vi "Big_LED_control.vi"() -> ()   [LabVIEW 2018]
uses:
  AT lib/AmateurStepperMotor.dll
  <instrlib>/niDMM/nidmm.llb/niDMM Function.ctl
  <instrlib>/niDMM/nidmm.llb/niDMM Resolution in Digits.ctl
  <instrlib>/niDCPower/nidcpower.llb/niDCPower Measurement Type.ctl
  <vilib>/Instr/_visa.llb/VISA Configure Serial Port (Instr).vi
  <instrlib>/niDMM/nidmm.llb/niDMM Configure Measurement Digits.vi
panel:
  out "IsOpen":bool
  out "Enum":enum16{"Exit", "4", "Промер", "2", "1"}(ring)
  in  "Tab Control":T1(tab)=enum."Сила света"
  in  "POWER":bool
  in  "Стоп":bool=TRUE
  in  "Resource Name":refnum<k15>="PXI1Slot2" caption="Источник питания"
  in  "Амперметр":refnum<k15>="PXI1Slot4" caption="NI DMM 1"
  in  "V_MB, V":dbl=5.0 caption="voltage level" format="%_6p"
  in  "curlim_V_MB, A":dbl=0.3 caption="current limit" format="%_6p"
  in  "curlim_V_RESERVE, A":dbl=0.1 caption="current limit" min=0.01 format="%_6p"
  out "currentmes_V_MB, A":dbl=-0.001986406197333734 caption="measurement" format="%_6g"
  out "currentmes_V_RESERVE, A":dbl=4.286668577189643e-07 caption="measurement" format="%_6g"
  in  "V_RESERVE, V":dbl caption="voltage level" format="%_6p"
  out "chart_2":dbl(graph)=4.286668577189643e-07
  out "chart_0":dbl(graph)=-0.001986406197333734 caption="Waveform Chart 5"
  in  "curlim_V_LED, A":dbl=0.01 caption="current limit" min=0.01 format="%_6p"
  in  "V_LED, V":dbl=2.000000000000001 caption="voltage level" format="%_6p"
  out "chart_1":dbl(graph)=9.464711192498274e-07 caption="Waveform Chart 5"
  out "currentmes_V_LED, A":dbl=9.464711192498274e-07 caption="measurement" format="%_6g"
  in  "NI DMM 1 Current Range 3":string(combo)="1" caption="Range"
  in  "NI DMM 1 units 3":string(combo)="1000" caption="Units"
  out "Current Char":dbl(graph)=0.008323229849338531
  out "Current":dbl=0.008323229849338531 format="%_6g"
  in  "Arduino":refnum<visa-resource-name>="COM14"
  in  "Сегменты":bool[](array[boolean])=[FALSE, FALSE, FALSE, FALSE, FALSE, FALSE, FALSE, FALSE, FALSE, FALSE, FALSE, FALSE, FALSE, FALSE, FALSE, FALSE, FALSE, FALSE]
  in  "Вольтметр":refnum<k15>="PXI1Slot5" caption="NI DMM 1"
  in  "NI DMM 1 Voltage Range 4":string(combo)="-1" caption="Range"
  out "Voltage Char":dbl(graph)=nan
  in  "NI DMM 1 units 4":string(combo)="1" caption="Units"
  out "Voltage":dbl=nan format="%_6g"
  out "Тип индикатора":string="Anode"
  in  "set pos":bool
  in  "new pos":dbl
  in  "Промер":bool caption="Промер сегмента"
  in  "Ophir 1 Info":u16(ring)=1 caption="Info" items=["Device : JUNO; s/n:903793", "Head : PD300R-3W   ; s/n:779628"]
  out "Ophir 1 Initialization":bool=TRUE caption="Initialization"
  out "Position":dbl
  out "Готово":bool
  in  "Стоп GoTo":bool
  in  "Погнали!":bool
  in  "Speed":dbl=1000.0
  in  "StepDivisor":i32(ring)=8 items=["D1"=1, "D2"=2, "D4"=4, "D8"=8, "D16"=16, "D32"=32]
  in  "StepMultiplicationFactor":dbl=1.0
  in  "Ophir 1 Wait":u32=100 caption="Wait"
  in  "Ophir 1 Clear":bool caption="Clear"
  out "Ophir 1 MAX":dbl=0.060000000000000005 caption="MAX" format="%#_5g"
  out "Ophir 1 Optical Power":dbl=0.060000000000000005 caption="Power" format="%#_4g"
  out "Ophir 1 Over Range":bool caption="Over Range"
  in  "Ophir 1 units":string(combo)="1000" caption="Units"
  in  "HoldOn":bool
  in  "AccelerationTime, s":dbl
  in  "DecelerationTime, s":dbl
  out "Ophir 1 Char":dbl(graph)=0.060000000000000005
  in  "Go To":dbl
  in  "wave_lenght":string="600"
  in  "Port Name":string="COM1"
  in  "measure path":path=path "D:/NI LabVIEW/MultiOpto/MultiOpto_1.2/Logs/SEL"
  in  "Сегмент":string="-" caption="Введи сегмент"
  in  "Температура":string="-" caption="Введи температуру"
  out "Образец №":string="0"
  in  "milliseconds to wait":u32=1000
  out "Разряд":dbl
  out "+/-":bool
  out "Power off":bool=TRUE
  in  "Ophir 1 error in (no error)":errorcluster caption="error in (no error)"
  out "Ophir 1 error out":errorcluster caption="error out"
  in  "Ophir 1 Select Communication Protocol":u16(ring) caption="Select Communication Protocol" items=["USB", "RS232", "GPIB"]
  in  "Ophir 1 Port Number (default 2)":i16=1 caption="Port Number (default 2)" min=0 max=20
  in  "Ophir 1 GPIB Address (10)":string="10" caption="GPIB Address (10)"
  out "Ophir 1 Real Optical Power":dbl=6e-05 format="%.6e"
  in  "Ophir 1 Baud Rate (3:9600)":i16(ring)=3 caption="Baud Rate (3:9600)" items=["300", "1200", "4800", "9600", "19200", "38400"]
  out "Ophir 1 dup Visa Session":refnum<visa-resource-name>="USB0::0x0BD3::0x0777::NI-VISA-40004::RAW" caption="dup Visa Session"
  in  "Ophir 1 usb channel":i16 caption="usb channel"
  in  "Command":string="Anode"
  in  "Записать":bool
  out "measure output file refnum":refnum<file>
  out "Device Response":string="*\n"
  out "Voltage, V":dbl=nan caption="Measurement" format="%.5f"
  out "Current, A":dbl=8.323229849338531e-06 caption="Measurement" format="%.5f"
  # "V_MB 5 В\nогрничение 300 м\n\nV_LED 2,1 В\nограничение 200 м"
  # "единицы мА\nrange 1 А"
  # "единицы В\nrange AUTO"
  # "24.063\n\n     I          U\n20 мА  1.3 В\n20 мА  1.4 В\n 7 мА   1.15 В"
  # "24.064\n\n     I          U\n10 мА  2 В\n10 мА  2.15 В\n 7 мА   1.9 В"
  # "Р1:  +25°C\nР2:  - 60°C\nР3:  +85°C"
  # "j"
  # "c"
  # "d"
  # "e"
  # "g"
  # "h"
  # "a"
  # "b"
  # "f"
  # "k"
  # "L"
  # "m"
  # "n"
  # "p"
  # "dp"
  # "all"
  # "необходимо выдерживать 1 с между нажатиями кнопок"
  # "Шаговик"
  # "Офир"
  # "это значение абсолютное"
  # "0. ввести номер образца\n1. включить нужный сегмент\n2. ввести его в поле справа\n3. вести температуру в поле слева\n4. нажать кнопку \"промер сегмента\""
  # "Введи ->"
  # "\"опрашивать кнопки не чаще, чем раз в секунду. сейчас кликать можно чаще, они загорятся, но ничего не произойдет\""
  # "Офир"
  # "автоматизировать подбор напряжения по известному максимальному напряжению и току. ОС по току сегмента"
  # "регклировка суммарного тока через индикатор"
  # "регулировать ток в зависимости от температуры.\nс ростом температуры растет ток.\nпид-регулятор??"
  # "1. каждый сегмент включаем по отдельности, резистором постраиваем ток до 10 мА\n2. напряжение V_LED при этом не меняется\n3. в такоом положении промеряем сегменты по отдельности\n4. для промера всего индикатора сразу подстраиваем напряжение при неизменном положении резисторов\n5. ток всех индикаторов = ток одного сегмента (10 мА) * число сегментов (15)\n6. добиваемся этого увеличением V_LED"
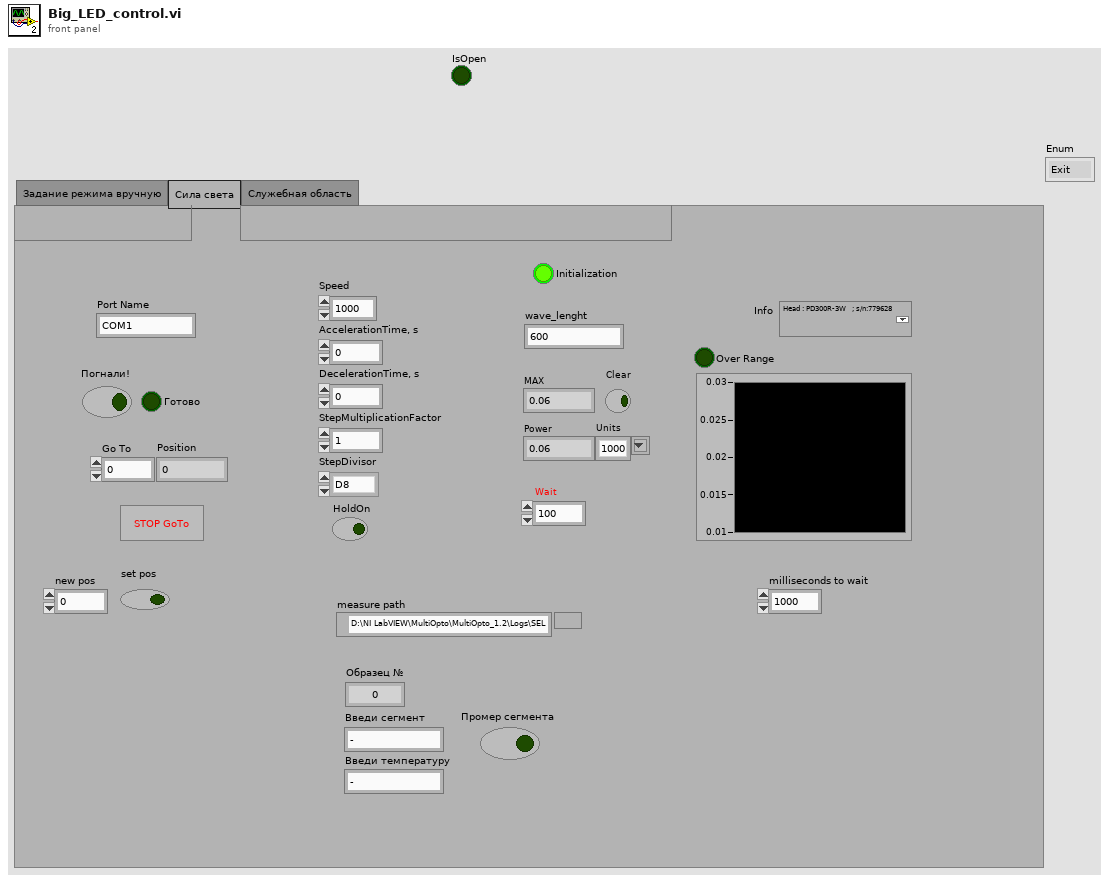
[diagram p1: front panel]
types:
  T1 = enum32{"Задание режима вручную", "Сила света", "Служебная область"}
  T2 = enum16{"open", "replace", "create", "open or create", "replace or create", "replace or create with confirmation"}
  T3 = typedef "niDCPower Measurement Type.ctl" = i32
  T4 = typedef "niDMM Function.ctl" = enum16{"DC Volts", "AC Volts", "DC Current", "AC Current", "2-wire Resistance", "4-wire Resistance", "Diode", "Frequency", "Period", "AC Volts DC Coupled", "Capacitance", "Inductance", "Temperature"}
  T5 = typedef "niDMM Resolution in Digits.ctl" = dbl
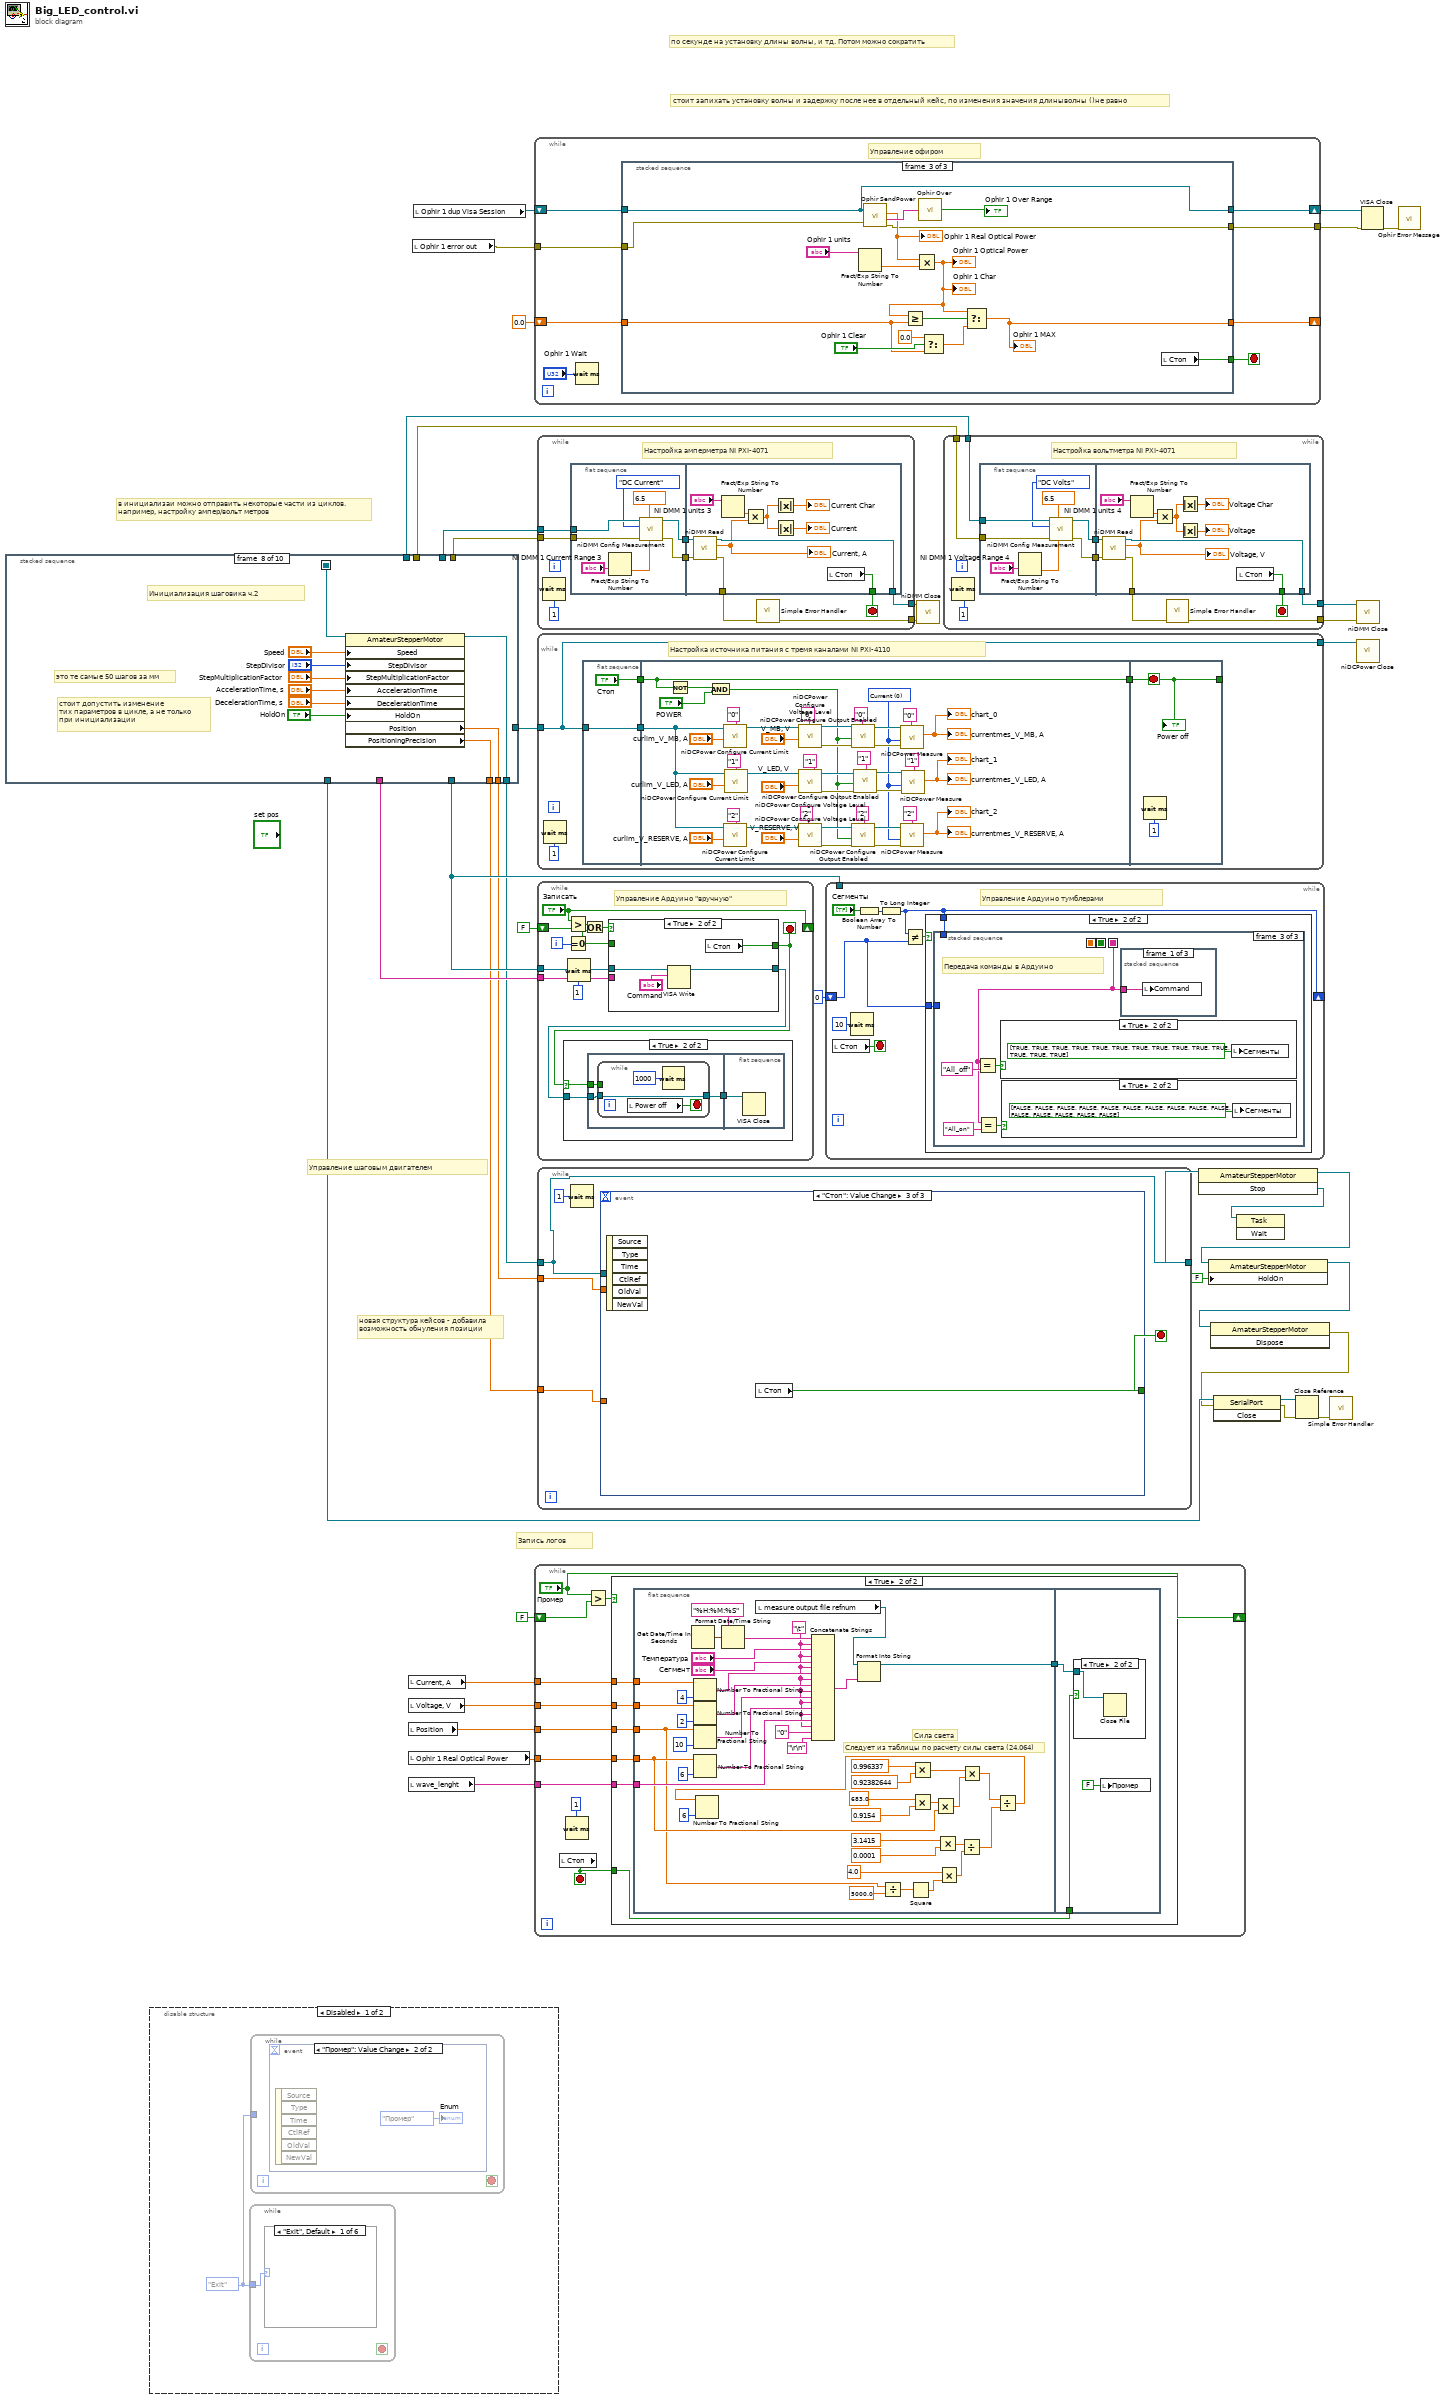
[diagram p0: block diagram]
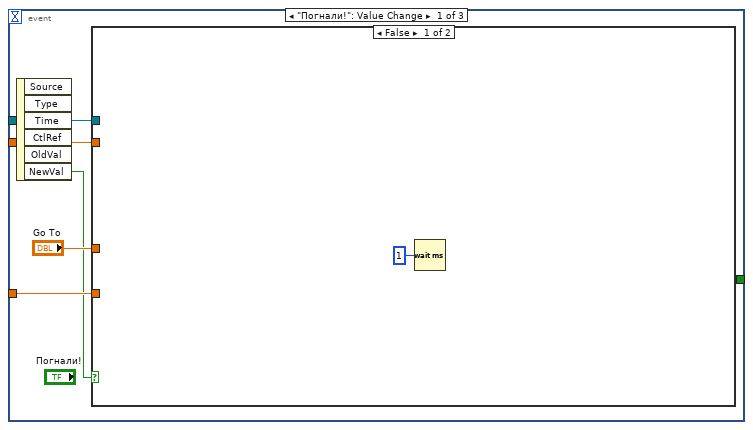
[diagram p2: hidden frame]
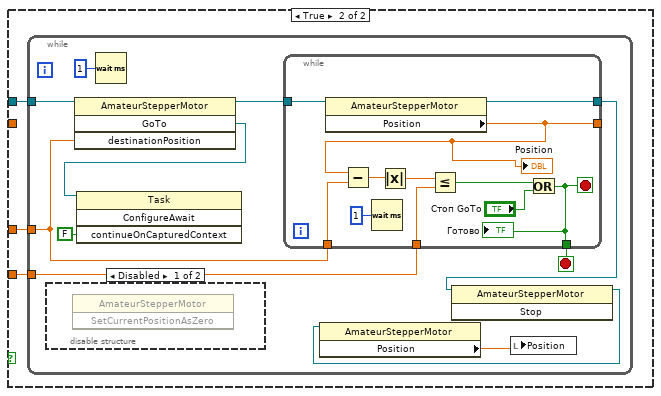
[diagram p3: hidden frame]
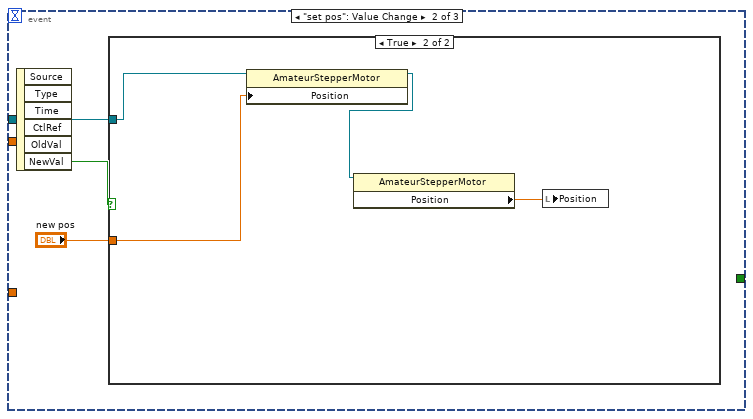
[diagram p5: hidden frame]
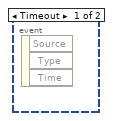
[diagram p12: hidden frame]
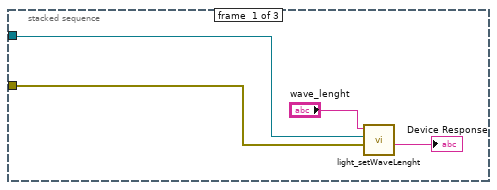
[diagram p16: hidden frame]
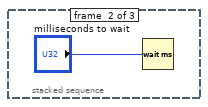
[diagram p17: hidden frame]
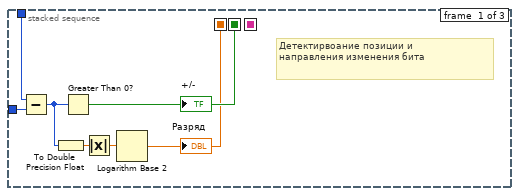
[diagram p19: hidden frame]
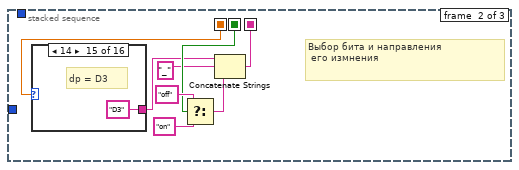
[diagram p20: hidden frame]
diagram:
  # "новая структура кейсов - добавила\nвозможность обнуления позиции"
  # "Управление шаговым двигателем"
  # "Запиcь логов"
  # "в инициализаи можно отправить некоторые части из циклов.\nнапример, настройку ампер/вольт метров"
  # "стоит запихать установку волны и задержку после нее в отдельный кейс, по изменения значения длиныволны ()не равно"
  # "по секунде на установку длины волны, и тд. Потом можно сократить"
  n1 = stacked-sequence {
    seq-local: [_ _ _ _ _ _ w91 _ _ _] -> [_ _ _ _ _ _ _ w100 _ _]
    tunnel: [_ _ _ w52 _ _ _ _ _ _] -> w27
    tunnel: [_ w48 _ _ _ _ _ _ _ _] -> w39
    tunnel: [_ w47 _ _ _ _ _ _ _ _] -> w38
    tunnel: [_ _ _ _ w58 _ _ _ _ _] -> w35
    tunnel: [_ _ _ _ _ _ _ _ _ w136] -> w34
    tunnel: [_ _ w51 _ _ _ _ _ _ _] -> w33
    tunnel: [_ _ w50 _ _ _ _ _ _ _] -> w32
    tunnel: [_ _ _ _ _ _ _ w103 _ _] -> w26
    tunnel: [_ _ _ _ _ _ _ w101 _ _] -> w24
    tunnel: [_ _ _ _ _ _ _ w102 _ _] -> w25
    tunnel: [_ _ _ _ _ _ w81 _ _ _] -> w18
    frame #0 {
      w41 = "-" ("Температура")
      w42 = 0.0 ("currentmes_2")
      w43 = FALSE ("Стоп")
      # "Обнуление переменных"
      n2 = local write "POWER"(w43) -> ()
      n3 = local write "Стоп"(w43) -> ()
      n4 = local write "+/-"(w43) -> ()
      n5 = local write "Погнали!"(w43) -> ()
      n6 = local write "Готово"(w43) -> ()
      n7 = local write "Стоп GoTo"(w43) -> ()
      n8 = local write "Go To"(w42) -> ()
      n9 = local write "currentmes_V_MB, A"(w42) -> ()
      n10 = local write "currentmes_V_LED, A"(w42) -> ()
      n11 = local write "currentmes_V_RESERVE, A"(w42) -> ()
      n12 = local write "Current"(w42) -> ()
      n13 = local write "Разряд"(w42) -> ()
      n14 = local write "Сегменты"(bool[] [FALSE, FALSE, FALSE, FALSE, FALSE, FALSE, FALSE, FALSE, FALSE, FALSE, FALSE, FALSE, FALSE, FALSE, FALSE, FALSE, FALSE, FALSE] ("Сегменты")) -> ()
      n15 = local write "Температура"(w41) -> ()
      n16 = local write "Command"("zero" ("Command 2")) -> ()
      n17 = local write "Сегмент"(w41) -> ()
      "Образец №" <- "0" ("Образец №")
    }
    frame #1 {
      # "Инициализация амперметра"
      n18 = call <instrlib>:"niDMM Initialize.vi"("Instrument Descriptor"="Амперметр") -> ("error out"=w48:errorcluster, "instrument handle out"=w47:refnum<k15>)  [unwired: 9 in]
    }
    frame #2 {
      # "Инициализация вольтметра"
      n19 = call <instrlib>:"niDMM Initialize.vi"("Instrument Descriptor"="Вольтметр") -> ("error out"=w50:errorcluster, "instrument handle out"=w51:refnum<k15>)  [unwired: 9 in]
    }
    frame #3 {
      # "Инициализация источника питания"
      n20 = call <instrlib>:"niDCPower Initialize.vi"("resource name"="Resource Name") -> ("error out"=w54:errorcluster, "instrument handle out"=w55:refnum<k15>)  [unwired: 3 in, 6 out]
      n21 = call <instrlib>:"niDCPower Configure Voltage Level.vi"("error in (no error)"=w54, "voltage level"=0.0, "channel name"="0,1,2", "instrument handle"=w55) -> ("instrument handle out"=w52:refnum<k15>)  [unwired: 6 in, 1 out]
    }
    frame #4 {
      # "Инициализация Ардуино"
      n22 = call-poly "VISA Configure Serial Port"("VISA resource name"="Arduino", "baud rate (9600)"=u32 9600) -> ("VISA resource name out"=w58:refnum<visa-resource-name>)  [unwired: 12 in, 1 out]
    }
    frame #5 {
      # "Инициализация офира"
      n23 = call "Ophir InitCom.vi"("GPIB Address (default 10)"="Ophir 1 GPIB Address (10)", "Communication (default USB 0)"="Ophir 1 Select Communication Protocol", "USB Channel number (default 0)"="Ophir 1 usb channel", "Port Number (default 2)"="Ophir 1 Port Number (default 2)", "error in (no error)"="Ophir 1 error in (no error)", "Baud Rate (3:9600)"="Ophir 1 Baud Rate (3:9600)") -> ("dup Visa Session"=w67:refnum<visa-resource-name>, "error out"=w66:errorcluster)  [unwired: 1 out]
      n24 = call "Ophir InstrInfo.vi"("Visa Session"=w67, "error in (no error)"=w66) -> ("dup Visa Session"=w79:refnum<visa-resource-name>, "Instrument Info"=w61:string, "error out"=w77:errorcluster)
      n25 = call "Ophir HeadInfo.vi"("Visa Session"=w79, "error in (no error)"=w77) -> ("error out"=w76:errorcluster, "dup Visa Session"=w78:refnum<visa-resource-name>, "Head Info"=w75:string)  [unwired: 6 out]
      n26 = call "Ophir InfoStrings.vi"("error in (no error)"=w76, "Head Info"=w75, "Instrument Info"=w61) -> ("error out"=w74:errorcluster, "Strings Array"=w73:string[])
      n27 = property on="Ophir 1 Info" class="Ring (strict)"("Strings []"=w73) -> ()  [unwired: 2 in, 2 out]
      n28 = call "Ophir ConfigDevice.vi"("Visa Session"=w78, "Measure Choice (0:Power)"=u16 0, "error in (no error)"=w74) -> ("dup Visa Session"=→"Ophir 1 dup Visa Session":refnum<visa-resource-name>, "OK ?"=→"Ophir 1 Initialization":bool, "error out"=→"Ophir 1 error out":errorcluster)  [unwired: 1 out]
    }
    frame #6 {
      w85 = 100 ("WriteTimeout")
      w90 = 1 items=["None", "One", "Two", "OnePointFive"] ("stopBits")
      w87 = 0 items=["None", "Odd", "Even", "Mark", "Space"] ("parity")
      # "убрали открытие порта. шаговик его и так сам откроет"
      # "Инициализация шаговика ч.1"
      n29 = constructor class="SerialPort"("portName"="Port Name", "baudRate"=57600, "parity"=w87, "dataBits"=8, "stopBits"=w90) -> (reference out=w84:refnum<k24>, error out=w83:errorcluster)  [unwired: 3 in, 6 out]
      n30 = property class="SerialPort"(reference=w84, error in=w83, "WriteTimeout"=w85, "ReadTimeout"=w85) -> (reference out=w81:refnum<k24>)  [unwired: 1 out]
      n31 = constructor class="AmateurStepperMotor"("serialPort"=w81) -> (reference out=w91:refnum<k24>, error out=w82:errorcluster)  [unwired: 3 in, 2 out]
      n32 = flat-sequence {
        tunnel: w82 -> [_]
        tunnel: w81 -> [w93]
        frame #0 {
          n33 = property class="SerialPort"(reference=w93) -> ("IsOpen"=→"IsOpen":bool)  [unwired: 1 in, 2 out]
        }
      }
    }
    frame #7 {
      # "стоит допустить изменение\nтих параметров в цикле, а не только \nпри инициализации"
      # "это те самые 50 шагов за мм"
      # "Инициализация шаговика ч.2"
      n34 = property class="AmateurStepperMotor"(reference=w100, "Speed"="Speed", "StepDivisor"="StepDivisor", "StepMultiplicationFactor"="StepMultiplicationFactor", "AccelerationTime"="AccelerationTime, s", "DecelerationTime"="DecelerationTime, s", "HoldOn"="HoldOn") -> (reference out=w103:refnum<k24>, "Position"=w101:dbl, "PositioningPrecision"=w102:dbl)  [unwired: 1 in, 1 out]
    }
    frame #8 {
      w106 = "\t"
      # "Инициализация логов"
      n35 = local read "Образец №"() -> (w130:string)
      n36 = Get Date/Time In Seconds() -> (seconds since 1Jan1904=w124:timestamp)
      n37 = Build Path(base path="measure path", name or relative path=w130) -> (appended path=w120:path)
      n38 = call <vilib>:"Check if File or Folder Exists.vi"("path"=w120) -> ("file or folder exists?"=w121:bool, "dup path"=w122:path)  [unwired: 8 in, 1 out]
      n39 = Format Date/Time String(time format string (%c)="MES %d %m %y %H.%M.%S", seconds (now)=w124) -> (date/time string=w125:string)  [unwired: 1 in]
      n40 = case shown="False" w121 {
        tunnel: w122 -> [w134 w135]
        tunnel: [w133 w135] -> w123
        frame False {
          n41 = Create Folder(path (use dialog)=w134) -> (created path=w133:path)  [unwired: 2 in, 2 out]
        }
        frame True {
        }
      }
      n42 = Concatenate Strings(w125, ".xls" ("string")) -> (w126:string)
      n43 = Build Path(base path=w123, name or relative path=w126) -> (appended path=w127:path)
      n44 = Open/Create/Replace File(file path (use dialog)=w127, operation (0:open)=T2."open or create", access (0:read/write)=enum16{"read/write", "read-only", "write-only"}."read/write") -> (refnum out=w128:refnum<file>)  [unwired: 3 in, 2 out]
      n45 = Set File Position(refnum=w128, from (0:start)=enum16{"start", "end", "current"}."end") -> (refnum out=w131:refnum<file>)  [unwired: 2 in, 1 out]
      n46 = Format Into String(initial string=w131, "Time" ("string"), w106, "Temperature, C" ("string"), w106, "Segment" ("string"), w106, "Current, mA" ("string"), w106, "Voltage, V" ("input 7"), w106, "Distance, m" ("string"), w106, "Power, W " ("string"), w106, "Wavelenght, nm" ("input 17"), w106, "Candlepower, kd" ("string"), "\r\n") -> (resulting string=→"measure output file refnum":refnum<file>)  [unwired: 2 in, 1 out]
    }
    frame #9 {
      # "Begin VI: ОК или ОА?"
      n47 = call "Begin.vi"() -> ("String"=w136:string)  [unwired: 8 in]
      "Тип индикатора" <- w136
      n48 = local write "Command"(w136) -> ()
    }
  }
  n49 = disable-structure shown="Disabled" {
    frame Disabled {
      w137 = enum16{"Exit", "4", "Промер", "2", "1"}."Exit"
      n50 = while {
        tunnel: w137 -> [w138]
        stop <- _ stop-if-true
        n51 = case shown="\"Exit\", Default" w138 {
          frame "Exit", Default {
          }
          frame "4" {
          }
          frame "2" {
          }
          frame "2" {
          }
          frame "1" {
          }
          frame "Промер" {
          }
        }
      }
      n52 = while {
        tunnel: w137 -> [_]
        stop <- _ stop-if-true
        n53 = event shown="[1] \"Промер\": Value Change" {
          selector: _ -> [_ _]
          dyn-events: _ -> [_ _]
          timeout: _ -> [_ _]
          event Timeout {
            n54 = event-data() -> ()  [unwired: 1 in, 3 out]
          }
          event "Промер": Value Change {
            n55 = event-data() -> ()  [unwired: 1 in, 6 out]
            "Enum" <- enum16{"Exit", "4", "Промер", "2", "1"}."Промер" ("Enum")
          }
        }
      }
    }
    frame Enabled {
    }
  }
  n56 = local read "Current, A"() -> (w17:dbl)
  n57 = local read "Voltage, V"() -> (w16:dbl)
  n58 = local read "Position"() -> (w15:dbl)
  n59 = local read "Ophir 1 Real Optical Power"() -> (w14:dbl)
  n60 = local read "wave_lenght"() -> (w13:string)
  n61 = local read "Ophir 1 error out"() -> (w22:errorcluster)
  n62 = local read "Ophir 1 dup Visa Session"() -> (w23:refnum<visa-resource-name>)
  n63 = while {
    tunnel: w17 -> [w149]
    tunnel: w16 -> [w148]
    tunnel: w15 -> [w147]
    tunnel: w14 -> [w146]
    tunnel: w13 -> [w145]
    shift-right: ["Промер"] -> _
    shift-left: FALSE ("Промер сегмента") -> [w142]
    stop <- w140 stop-if-true
    n64 = local read "Стоп"() -> (w140:bool)
    n65 = Wait (ms)(milliseconds to wait=u32 1) -> ()  [unwired: 1 out]
    n66 = Greater?(x="Промер", y=w142) -> (0:w143:bool)
    n67 = case shown="True" w143 {
      tunnel: w149 -> [_ w156]
      tunnel: w148 -> [_ w155]
      tunnel: w147 -> [_ w152]
      tunnel: w146 -> [_ w153]
      tunnel: w145 -> [_ w154]
      tunnel: w140 -> [_ w150]
      frame False {
      }
      frame True {
        n68 = flat-sequence {
          tunnel: w156 -> [w189]
          tunnel: w155 -> [w188]
          tunnel: w154 -> [w186]
          tunnel: w153 -> [w176]
          tunnel: w152 -> [w166]
          tunnel: [w158] -> w151
          tunnel: w151 -> [w202]
          tunnel: w150 -> [w201]
          frame #0 {
            w185 = "\t"
            # "Сила света"
            # "Следует из таблицы по расчету силы света (24.064)"
            n69 = Get Date/Time In Seconds() -> (seconds since 1Jan1904=w199:timestamp)
            n70 = Number To Fractional String(number=w189, precision (6)=i16 4) -> (F-format string=w192:string)  [unwired: 2 in]
            n71 = Number To Fractional String(number=w188, precision (6)=i16 2) -> (F-format string=w191:string)  [unwired: 2 in]
            n72 = Number To Fractional String(number=w166, precision (6)=i16 10) -> (F-format string=w190:string)  [unwired: 2 in]
            n73 = Number To Fractional String(number=w176, precision (6)=i16 6) -> (F-format string=w187:string)  [unwired: 2 in]
            n74 = Format Date/Time String(time format string (%c)="%H:%M:%S", seconds (now)=w199) -> (date/time string=w197:string)  [unwired: 1 in]
            n75 = local read "measure output file refnum"() -> (w193:refnum<file>)
            n76 = Concatenate Strings(w197, w185, "Температура", w185, "Сегмент", w185, w192, w185, w191, w185, w190, w185, w187, w185, w186, w185, "0" ("string"), "\r\n") -> (w194:string)
            n77 = Format Into String(initial string=w193, w194) -> (resulting string=w158:refnum<file>)  [unwired: 2 in, 1 out]
            n78 = Divide(x=w166, y=5000.0) -> (x/y=w168:dbl)
            n79 = Square(x=w168) -> (x^2=w167:dbl)
            n80 = Multiply(x=0.996337, y=0.92382644) -> (x*y=w181:dbl)
            n81 = Multiply(x=683.0, y=0.9154) -> (x*y=w177:dbl)
            n82 = Multiply(x=w177, y=w176) -> (x*y=w175:dbl)
            n83 = Multiply(x=3.1415, y=0.0001) -> (x*y=w171:dbl)
            n84 = Multiply(x=4.0, y=w167) -> (x*y=w170:dbl)
            n85 = Divide(x=w171, y=w170) -> (x/y=w172:dbl)
            n86 = Multiply(x=w181, y=w175) -> (x*y=w180:dbl)
            n87 = Divide(x=w180, y=w172) -> (x/y=w164:dbl)
            n88 = Number To Fractional String(number=w164, precision (6)=i16 6) -> ()  [unwired: 2 in, 1 out]
          }
          frame #1 {
            n89 = case shown="True" w201 {
              tunnel: w202 -> [_ w203]
              frame False {
              }
              frame True {
                n90 = Close File(refnum=w203) -> ()  [unwired: 1 in, 2 out]
              }
            }
            n91 = local write "Промер"(FALSE ("Промер")) -> ()
          }
        }
      }
    }
  }
  n92 = while {
    tunnel: w22 -> [w210]
    shift-right: [w206] -> _
    shift-left: 0.0 ("t") -> [w209]
    shift-right: [w207] -> w11
    shift-left: w23 -> [w211]
    tunnel: [w205] -> w10
    stop <- w204 stop-if-true
    # "Управление офиром"
    n93 = Wait (ms)(milliseconds to wait="Ophir 1 Wait") -> ()  [unwired: 1 out]
    n94 = stacked-sequence {
      tunnel: w211 -> [w215 _ w218]
      tunnel: w210 -> [w214 _ w220]
      tunnel: w209 -> [_ _ w221]
      tunnel: [_ _ w218] -> w207
      tunnel: [_ _ w222] -> w206
      tunnel: [_ _ w219] -> w205
      tunnel: [_ _ w217] -> w204
      frame #0 {
        n95 = call "light_setWaveLenght.vi"("error in (no error)"=w214, "Visa Session"=w215, "wave_lenght"="wave_lenght") -> ("Device Response"=→"Device Response":string)  [unwired: 6 in, 2 out]
      }
      frame #1 {
        n96 = Wait (ms)(milliseconds to wait="milliseconds to wait") -> ()  [unwired: 1 out]
      }
      frame #2 {
        n97 = Fract/Exp String To Number(string="Ophir 1 units") -> (number=w225:dbl)  [unwired: 3 in, 1 out]
        n98 = call "Ophir SendPower.vi"("Visa Session"=w218, "error in (no error)"=w220) -> ("Value Number"=w224:dbl, "Value String"=w231:string, "error out"=w219:errorcluster)  [unwired: 1 out]
        "Ophir 1 Real Optical Power" <- w224
        n99 = Multiply(x=w224, y=w225) -> (x*y=w228:dbl)
        "Ophir 1 Char" <- w228
        "Ophir 1 Optical Power" <- w228
        n100 = Greater Or Equal?(x=w228, y=w221) -> (x >= y?=w229:bool)
        n101 = call "Ophir Over.vi"("Value String"=w231) -> ("Overrange"=→"Ophir 1 Over Range":bool)
        n102 = Select(t=0.0, s="Ophir 1 Clear", f=w221) -> (s? t:f=w227:dbl)
        n103 = Select(t=w228, s=w229, f=w227) -> (s? t:f=w222:dbl)
        "Ophir 1 MAX" <- w222
        n104 = local read "Стоп"() -> (w217:bool)
      }
    }
  }
  n105 = while {
    tunnel: w27 -> [w234]
    tunnel: [w234] -> w36
    stop <- w235 stop-if-true
    # "Настройка источника питания с тремя каналами NI PXI-4110"
    n106 = Wait (ms)(milliseconds to wait=u32 1) -> ()  [unwired: 1 out]
    n107 = flat-sequence {
      tunnel: w234 -> [w240]
      tunnel: [w240] -> w237
      tunnel: ["Стоп"] -> w236
      tunnel: w237 -> [w248]
      tunnel: w236 -> [w282]
      tunnel: [w282] -> w233
      tunnel: [w284] -> w235
      tunnel: w233 -> [w284]
      frame #0 {
      }
      frame #1 {
        w247 = T3 0 items=["Current", "Voltage"] ("measurement type")
        n108 = Not(x=w282) -> (.not. x?=w281:bool)
        n109 = And(x=w281, y="POWER") -> (x .and. y?=w243:bool)
        n110 = call <instrlib>:"niDCPower Configure Current Limit.vi"("current limit"="curlim_V_MB, A", "channel name"="0", "instrument handle"=w248) -> ("instrument handle out"=w267:refnum<k15>)  [unwired: 7 in, 1 out]
        n111 = call <instrlib>:"niDCPower Configure Current Limit.vi"("current limit"="curlim_V_RESERVE, A", "channel name"="2", "instrument handle"=w248) -> ("instrument handle out"=w266:refnum<k15>)  [unwired: 7 in, 1 out]
        n112 = call <instrlib>:"niDCPower Configure Current Limit.vi"("current limit"="curlim_V_LED, A", "channel name"="1", "instrument handle"=w248) -> ("instrument handle out"=w275:refnum<k15>)  [unwired: 7 in, 1 out]
        n113 = call <instrlib>:"niDCPower Configure Voltage Level.vi"("voltage level"="V_MB, V", "channel name"="0", "instrument handle"=w267) -> ("error out"=w272:errorcluster, "instrument handle out"=w269:refnum<k15>)  [unwired: 7 in]
        n114 = call <instrlib>:"niDCPower Configure Voltage Level.vi"("voltage level"="V_LED, V", "channel name"="1", "instrument handle"=w275) -> ("error out"=w278:errorcluster, "instrument handle out"=w276:refnum<k15>)  [unwired: 7 in]
        n115 = call <instrlib>:"niDCPower Configure Voltage Level.vi"("voltage level"="V_RESERVE, V", "channel name"="2", "instrument handle"=w266) -> ("error out"=w271:errorcluster, "instrument handle out"=w270:refnum<k15>)  [unwired: 7 in]
        n116 = call <instrlib>:"niDCPower Configure Output Enabled.vi"("error in (no error)"=w272, "output enabled"=w243, "channel name"="0", "instrument handle"=w269) -> ("error out"=w262:errorcluster, "instrument handle out"=w263:refnum<k15>)  [unwired: 6 in]
        n117 = call <instrlib>:"niDCPower Configure Output Enabled.vi"("error in (no error)"=w271, "output enabled"=w243, "channel name"="2", "instrument handle"=w270) -> ("error out"=w261:errorcluster, "instrument handle out"=w260:refnum<k15>)  [unwired: 6 in]
        n118 = call <instrlib>:"niDCPower Configure Output Enabled.vi"("error in (no error)"=w278, "output enabled"=w243, "channel name"="1", "instrument handle"=w276) -> ("error out"=w279:errorcluster, "instrument handle out"=w277:refnum<k15>)  [unwired: 6 in]
        n119 = call <instrlib>:"niDCPower Measure.vi"("error in (no error)"=w262, "measurement type"=w247, "channel name"="0", "instrument handle"=w263) -> ("measurement"=→"currentmes_V_MB, A" →"chart_0":dbl)  [unwired: 5 in, 2 out]
        n120 = call <instrlib>:"niDCPower Measure.vi"("error in (no error)"=w261, "measurement type"=w247, "channel name"="2", "instrument handle"=w260) -> ("measurement"=→"currentmes_V_RESERVE, A" →"chart_2":dbl)  [unwired: 5 in, 2 out]
        n121 = call <instrlib>:"niDCPower Measure.vi"("error in (no error)"=w279, "measurement type"=w247, "channel name"="1", "instrument handle"=w277) -> ("measurement"=→"chart_1" →"currentmes_V_LED, A":dbl)  [unwired: 5 in, 2 out]
      }
      frame #2 {
        n122 = Wait (ms)(milliseconds to wait=u32 1) -> ()  [unwired: 1 out]
        "Power off" <- w284
      }
    }
  }
  n123 = while {
    tunnel: w35 -> [w292]
    shift-right: ["Записать"] -> _
    shift-left: FALSE ("Записать") -> [w294]
    tunnel: w34 -> [w290]
    i -> [w291]
    stop <- w285 stop-if-true
    # "Управление Ардуино \"вручную\""
    n124 = Greater?(x="Записать", y=w294) -> (0:w288:bool)
    n125 = Equal To 0?(x=w291) -> (x = 0?=w287:bool)
    n126 = Wait (ms)(milliseconds to wait=u32 1) -> ()  [unwired: 1 out]
    n127 = Or(x=w288, y=w287) -> (x .or. y?=w289:bool)
    n128 = case shown="True" w289 {
      tunnel: w292 -> [w306 w311]
      tunnel: [w307 w310] -> w285
      tunnel: w290 -> [_ _]
      tunnel: w287 -> [_ _]
      tunnel: [w306 w308] -> w286
      frame False {
        n129 = local read "Стоп"() -> (w307:bool)
      }
      frame True {
        n130 = VISA Write(VISA resource name=w311, write buffer="Command") -> (VISA resource name out=w308:refnum<visa-resource-name>)  [unwired: 1 in, 2 out]
        n131 = local read "Стоп"() -> (w310:bool)
      }
    }
    n132 = case shown="True" w285 {
      selector: w285 -> [_ w296]
      tunnel: w286 -> [_ w298]
      frame False {
      }
      frame True {
        n133 = flat-sequence {
          tunnel: w298 -> [w301]
          tunnel: [w300] -> w297
          tunnel: w296 -> [w299]
          tunnel: w297 -> [w305]
          frame #0 {
            n134 = while {
              tunnel: w301 -> [w304]
              tunnel: [w304] -> w300
              tunnel: w299 -> [_]
              stop <- w302 stop-if-true
              n135 = local read "Power off"() -> (w302:bool)
              n136 = Wait (ms)(milliseconds to wait=u32 1000) -> ()  [unwired: 1 out]
            }
          }
          frame #1 {
            n137 = VISA Close(VISA resource name=w305) -> ()  [unwired: 1 in, 1 out]
          }
        }
      }
    }
  }
  n138 = while {
    tunnel: [w318] -> w28
    tunnel: w38 -> [w316]
    tunnel: w39 -> [w315]
    tunnel: [w312] -> w29
    stop <- w314 stop-if-true
    # "Настройка амперметра NI PXI-4071"
    n139 = Wait (ms)(milliseconds to wait=u32 1) -> ()  [unwired: 1 out]
    n140 = flat-sequence {
      tunnel: [w325] -> w320
      tunnel: w316 -> [w323]
      tunnel: w315 -> [w327]
      tunnel: [w324] -> w319
      tunnel: w320 -> [w336]
      tunnel: w319 -> [w339]
      tunnel: [w335] -> w314
      tunnel: [w334] -> w312
      tunnel: [w333] -> w313
      frame #0 {
        w321 = T5 6.5 items=["3 1/2"=3.5, "4 1/2"=4.5, "5 1/2"=5.5, "6 1/2"=6.5, "7 1/2"=7.5] ("Resolution in Digits")
        n141 = Fract/Exp String To Number(string="NI DMM 1 Current Range 3") -> (number=w326:dbl)  [unwired: 3 in, 1 out]
        n142 = call-poly <instrlib>:"niDMM Config Measurement.vi"("Range"=w326, "Resolution in Digits"=w321, "error in (no error)"=w327, "Function"=niDMM_Function."DC Current" ("Measurement Type"), "instrument handle"=w323) -> ("error out"=w324:errorcluster, "instrument handle out"=w325:refnum<k15>)  [unwired: 5 in]
      }
      frame #1 {
        n143 = call <instrlib>:"niDMM Read.vi"("error in (no error)"=w339, "instrument handle"=w336) -> ("error out"=w333:errorcluster, "Measurement"=w329:dbl, "instrument handle out"=w334:refnum<k15>)  [unwired: 7 in]
        "Current, A" <- w329
        n144 = Fract/Exp String To Number(string="NI DMM 1 units 3") -> (number=w337:dbl)  [unwired: 3 in, 1 out]
        n145 = Multiply(x=w337, y=w329) -> (x*y=w330:dbl)
        n146 = Absolute Value(x=w330) -> (abs(x)=→"Current Char":dbl)
        n147 = Absolute Value(x=w330) -> (abs(x)=→"Current":dbl)
        n148 = local read "Стоп"() -> (w335:bool)
      }
    }
    n149 = call <vilib>:"Simple Error Handler.vi"("error in (no error)"=w313) -> ("error out"=w318:errorcluster)  [unwired: 1 in, 7 out]
  }
  n150 = while {
    tunnel: w26 -> [w341]
    tunnel: w25 -> [w343]
    tunnel: [w341] -> w8
    tunnel: w24 -> [w344]
    stop <- w340 stop-if-true
    n151 = Wait (ms)(milliseconds to wait=u32 1) -> ()  [unwired: 1 out]
    n152 = event shown="[2] \"Стоп\": Value Change" {
      selector: _ -> [_ _ _]
      dyn-events: _ -> [_ _ _]
      timeout: _ -> [_ _ _]
      tunnel: w341 -> [w349 w377 _]
      tunnel: w344 -> [w348 _ _]
      tunnel: w343 -> [w347 _ _]
      tunnel: [_ _ w383] -> w340
      event "Погнали!": Value Change {
        n153 = event-data() -> ("NewVal"=w345:bool)  [unwired: 1 in, 5 out]
        n154 = case shown="False" w345 {
          tunnel: "Go To" -> [_ w353]
          tunnel: w349 -> [_ w352]
          tunnel: w348 -> [_ _]
          tunnel: w347 -> [_ w351]
          frame False {
            n155 = Wait (ms)(milliseconds to wait=u32 1) -> ()  [unwired: 1 out]
          }
          frame True {
            n156 = while {
              tunnel: w353 -> [w360]
              tunnel: w352 -> [w361]
              tunnel: w351 -> [w363]
              stop <- w364 stop-if-true
              n157 = disable-structure shown="Disabled" {
                frame Disabled {
                  n158 = invoke class="AmateurStepperMotor" method="SetCurrentPositionAsZero"() -> ()  [unwired: 3 in, 3 out]
                }
                frame Enabled {
                }
              }
              n159 = invoke class="AmateurStepperMotor" method="GoTo"(reference=w361, "destinationPosition"=w360) -> (reference out=w356:refnum<k24>, "GoTo"=w359:refnum<k24>)  [unwired: 2 in, 2 out]
              n160 = invoke class="Task" method="ConfigureAwait"(reference=w359, "continueOnCapturedContext"=FALSE) -> ()  [unwired: 2 in, 4 out]
              n161 = Wait (ms)(milliseconds to wait=u32 1) -> ()  [unwired: 1 out]
              n162 = while {
                tunnel: [w365] -> _
                tunnel: [w367] -> w357
                tunnel: [w369] -> w364
                tunnel: w360 -> [w374]
                tunnel: w363 -> [w372]
                tunnel: w356 -> [w366]
                stop <- w369 stop-if-true
                n163 = property class="AmateurStepperMotor"(reference=w366) -> (reference out=w367:refnum<k24>, "Position"=w365:dbl)  [unwired: 1 in, 1 out]
                "Position" <- w365
                n164 = Subtract(x=w365, y=w374) -> (x-y=w375:dbl)
                n165 = Wait (ms)(milliseconds to wait=u32 1) -> ()  [unwired: 1 out]
                n166 = Absolute Value(x=w375) -> (abs(x)=w373:dbl)
                n167 = Less Or Equal?(x=w373, y=w372) -> (x <= y?=w371:bool)
                n168 = Or(x=w371, y="Стоп GoTo") -> (x .or. y?=w369:bool)
                "Готово" <- w369
              }
              n169 = invoke class="AmateurStepperMotor" method="Stop"(reference=w357) -> (reference out=w355:refnum<k24>)  [unwired: 2 in, 2 out]
              n170 = property class="AmateurStepperMotor"(reference=w355) -> ("Position"=w354:dbl)  [unwired: 1 in, 2 out]
              n171 = local write "Position"(w354) -> ()
            }
          }
        }
      }
      event "set pos": Value Change {
        n172 = event-data() -> ("NewVal"=w378:bool)  [unwired: 1 in, 5 out]
        n173 = case shown="True" w378 {
          tunnel: w377 -> [_ w382]
          tunnel: "new pos" -> [_ w381]
          frame False {
          }
          frame True {
            n174 = property class="AmateurStepperMotor"(reference=w382, "Position"=w381) -> (reference out=w380:refnum<k24>)  [unwired: 1 in, 1 out]
            n175 = property class="AmateurStepperMotor"(reference=w380) -> ("Position"=w379:dbl)  [unwired: 1 in, 2 out]
            n176 = local write "Position"(w379) -> ()
          }
        }
      }
      event "Стоп": Value Change {
        n177 = event-data() -> ()  [unwired: 1 in, 6 out]
        n178 = local read "Стоп"() -> (w383:bool)
      }
    }
  }
  n179 = while {
    shift-right: [w386] -> _
    shift-left: 0 -> [w387]
    tunnel: w35 -> [_]
    stop <- w390 stop-if-true
    # "Управление Ардуино тумблерами"
    n180 = local read "Стоп"() -> (w390:bool)
    n181 = Wait (ms)(milliseconds to wait=u32 10 ("millisecond timer value")) -> ()  [unwired: 1 out]
    n182 = Boolean Array To Number(Boolean array="Сегменты") -> (number=w385:u32)
    n183 = To Long Integer(number=w385) -> (32bit integer=w386:i32)
    n184 = Not Equal?(x=w386, y=w387) -> (x != y?=w388:bool)
    n185 = case shown="True" w388 {
      tunnel: w386 -> [_ w391]
      tunnel: w387 -> [_ w392]
      frame False {
      }
      frame True {
        n186 = stacked-sequence {
          seq-local: [w395 _ _] -> [_ w405 _]
          seq-local: [w393 _ _] -> [_ w400 _]
          seq-local: [_ w401 _] -> [_ _ w425]
          tunnel: w391 -> [w397 _ _]
          tunnel: w392 -> [w396 _ _]
          frame #0 {
            # "Детектирвоание позиции и\nнаправления изменения бита"
            n187 = Subtract(x=w397, y=w396) -> (x-y=w398:i32)
            n188 = To Double Precision Float(number=w398) -> (double precision float=w399:dbl)
            n189 = Greater Than 0?(x=w398) -> (x > 0?=w395:bool)
            "+/-" <- w395
            n190 = Absolute Value(x=w399) -> (abs(x)=w394:dbl)
            n191 = Logarithm Base 2(1:w394) -> (0:w393:dbl)
            "Разряд" <- w393
          }
          frame #1 {
            # "Выбор бита и направления\n его измнения"
            n192 = case shown="14" w400 {
              tunnel: ["D10" "D9" "D5" "D8" "D11" "D12" "A1" "D4" "A5" "A4" "A3" "A2" "A0" "D13" "D3" "All"] -> w403
              frame 0, Default {
                # "a = D10"
              }
              frame 1 {
                # "b = D9"
              }
              frame 2 {
                # "c = D5"
              }
              frame 3 {
                # "d = D8"
              }
              frame 4 {
                # "e = D11"
              }
              frame 5 {
                # "f = D12"
              }
              frame 6 {
                # "g = A1"
              }
              frame 7 {
                # "h = D4"
              }
              frame 8 {
                # "j = A5"
              }
              frame 9 {
                # "k = A4"
              }
              frame 10 {
                # "L = A3"
              }
              frame 11 {
                # "m = A2"
              }
              frame 12 {
                # "n = A0"
              }
              frame 13 {
                # "p = D13"
              }
              frame 14 {
                # "dp = D3"
              }
              frame 15 {
              }
            }
            n193 = Select(t="off", s=w405, f="on") -> (s? t:f=w402:string)
            n194 = Concatenate Strings(w403, "_" ("string"), w402) -> (w401:string)
          }
          frame #2 {
            # "Передача команды в Ардуино"
            n195 = Equal?(x=w425, y="All_off") -> (x = y?=w428:bool)
            n196 = Equal?(x=w425, y="All_on") -> (x = y?=w426:bool)
            n197 = case shown="True" w428 {
              frame False {
              }
              frame True {
                n198 = local write "Сегменты"(bool[] [TRUE, TRUE, TRUE, TRUE, TRUE, TRUE, TRUE, TRUE, TRUE, TRUE, TRUE, TRUE, TRUE, TRUE, TRUE, TRUE] ("Сегменты")) -> ()
              }
            }
            n199 = case shown="True" w426 {
              frame False {
              }
              frame True {
                n200 = local write "Сегменты"(bool[] [FALSE, FALSE, FALSE, FALSE, FALSE, FALSE, FALSE, FALSE, FALSE, FALSE, FALSE, FALSE, FALSE, FALSE, FALSE, FALSE] ("Сегменты")) -> ()
              }
            }
            n201 = stacked-sequence {
              tunnel: w425 -> [w431 _ _]
              frame #0 {
                n202 = local write "Command"(w431) -> ()
              }
              frame #1 {
                n203 = local write "Записать"(TRUE ("Записать")) -> ()
                n204 = Wait (ms)(milliseconds to wait=u32 1000) -> ()  [unwired: 1 out]
              }
              frame #2 {
                n205 = local write "Записать"(FALSE ("Записать")) -> ()
                n206 = Wait (ms)(milliseconds to wait=u32 1000) -> ()  [unwired: 1 out]
              }
            }
          }
        }
      }
    }
  }
  n207 = call <instrlib>:"niDMM Close.vi"("error in (no error)"=w28, "instrument handle"=w29) -> ()  [unwired: 9 in, 1 out]
  n208 = while {
    tunnel: [w442] -> w30
    tunnel: w33 -> [w440]
    tunnel: w32 -> [w439]
    tunnel: [w436] -> w31
    stop <- w438 stop-if-true
    # "Настройка вольтметра NI PXI-4071"
    n209 = Wait (ms)(milliseconds to wait=u32 1) -> ()  [unwired: 1 out]
    n210 = flat-sequence {
      tunnel: [w449] -> w444
      tunnel: w440 -> [w447]
      tunnel: w439 -> [w451]
      tunnel: [w448] -> w443
      tunnel: w444 -> [w460]
      tunnel: w443 -> [w463]
      tunnel: [w459] -> w438
      tunnel: [w458] -> w436
      tunnel: [w457] -> w437
      frame #0 {
        w445 = T5 6.5 items=["3 1/2"=3.5, "4 1/2"=4.5, "5 1/2"=5.5, "6 1/2"=6.5, "7 1/2"=7.5] ("Resolution in Digits")
        n211 = Fract/Exp String To Number(string="NI DMM 1 Voltage Range 4") -> (number=w450:dbl)  [unwired: 3 in, 1 out]
        n212 = call-poly <instrlib>:"niDMM Config Measurement.vi"("Range"=w450, "Resolution in Digits"=w445, "error in (no error)"=w451, "Function"=niDMM_Function."DC Volts" ("Measurement Type"), "instrument handle"=w447) -> ("error out"=w448:errorcluster, "instrument handle out"=w449:refnum<k15>)  [unwired: 5 in]
      }
      frame #1 {
        n213 = call <instrlib>:"niDMM Read.vi"("error in (no error)"=w463, "instrument handle"=w460) -> ("error out"=w457:errorcluster, "Measurement"=w455:dbl, "instrument handle out"=w458:refnum<k15>)  [unwired: 7 in]
        "Voltage, V" <- w455
        n214 = Fract/Exp String To Number(string="NI DMM 1 units 4") -> (number=w461:dbl)  [unwired: 3 in, 1 out]
        n215 = Multiply(x=w461, y=w455) -> (x*y=w453:dbl)
        n216 = Absolute Value(x=w453) -> (abs(x)=→"Voltage Char":dbl)
        n217 = Absolute Value(x=w453) -> (abs(x)=→"Voltage":dbl)
        n218 = local read "Стоп"() -> (w459:bool)
      }
    }
    n219 = call <vilib>:"Simple Error Handler.vi"("error in (no error)"=w437) -> ("error out"=w442:errorcluster)  [unwired: 1 in, 7 out]
  }
  n220 = invoke class="AmateurStepperMotor" method="Stop"(reference=w8) -> (reference out=w6:refnum<k24>, "Stop"=w7:refnum<k24>)  [unwired: 2 in, 1 out]
  n221 = property class="AmateurStepperMotor"(reference=w6, "HoldOn"=FALSE) -> (reference out=w5:refnum<k24>)  [unwired: 1 in, 1 out]
  n222 = invoke class="AmateurStepperMotor" method="Dispose"(reference=w5) -> (error out=w2:errorcluster)  [unwired: 2 in, 2 out]
  n223 = invoke class="SerialPort" method="Close"(reference=w18, error in=w2) -> (reference out=w1:refnum<k24>, error out=w3:errorcluster)  [unwired: 1 in, 1 out]
  n224 = invoke class="Task" method="Wait"(reference=w7) -> ()  [unwired: 2 in, 3 out]
  n225 = Close Reference(reference=w1, error in (no error)=w3) -> (error out=w4:errorcluster)
  n226 = call <vilib>:"Simple Error Handler.vi"("error in (no error)"=w4) -> ()  [unwired: 1 in, 8 out]
  n227 = call <instrlib>:"niDMM Close.vi"("error in (no error)"=w30, "instrument handle"=w31) -> ()  [unwired: 9 in, 1 out]
  n228 = call <instrlib>:"niDCPower Close.vi"("instrument handle"=w36) -> ()  [unwired: 10 in, 1 out]
  n229 = VISA Close(VISA resource name=w11, error in (no error)=w10) -> (error out=w20:errorcluster)
  n230 = call "Ophir Error Message.vi"("error in (no error)"=w20) -> ()  [unwired: 3 in, 4 out]
